vi "Workspace.vi"() -> ()   [LabVIEW 2011]
panel:
  in  "Workspace":path
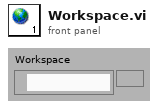
[diagram p1: front panel]
diagram:
